vi "OnDataChange.vi"(0 "Microscope Controller in":refnum<class "MicroscopeController.lvclass">, 1 "DataExchange":T1, 3 "error in (no error)":errorcluster) -> (7 "Microscope Controller out":refnum<class "MicroscopeController.lvclass">, 10 "error out":errorcluster)   [LabVIEW 2020]
uses:
  Model/Hardware Abstraction Layer/Component/Device/Device/DataExchange.ctl
  Interface/DataListener/DataListener.lvclass
  MicroscopeController.lvclass
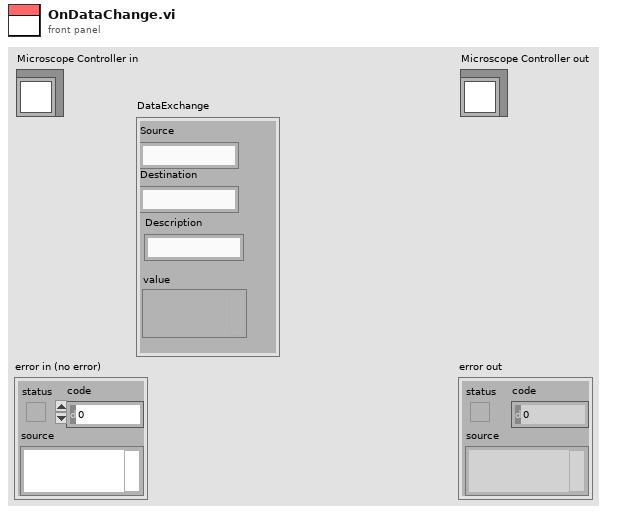
[diagram p1: front panel]
types:
  T1 = typedef "DataListener.lvclass/DataExchange.ctl" = cluster{"Source":string, "Destination":string, "Description":string, "value":variant}
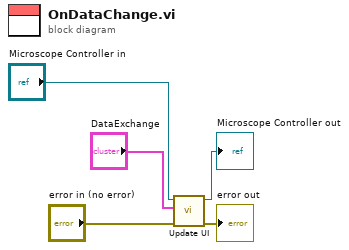
[diagram p0: block diagram]
diagram:
  n1 = call "Update UI.vi"("error in (no error)"="error in (no error)", "DataExchange"="DataExchange", "Microscope Controller in"="Microscope Controller in") -> ("error out"=→"error out":errorcluster, "Microscope Controller out"=→"Microscope Controller out":refnum<class "MicroscopeController.lvclass">)  [unwired: 7 in]
